vi "Incrementel Tester.vi"() -> ()   [LabVIEW 2013]
uses:
  <vilib>/Platform/TimedLoop/XDataNode/timing_clust.ctl
  <vilib>/Platform/TimedLoop/XDataNode/nitl_modes.ctl
  <vilib>/Platform/TimedLoop/XDataNode/wakeup.ctl
  <vilib>/rvi/Emulation/niFpgaSctlEmulationGetInTimedLoop.vi
  <vilib>/rvi/Emulation/niFpgaEmulationReportErrorSimple.vi
  <vilib>/rvi/Emulation/niFpgaGetClockAttributes.vi
  <vilib>/rvi/Emulation/niFpgaCriticalErrorInLSC.vi
  <vilib>/rvi/eio/common/nirviEmuTemplateMethod_errors.vi
  <vilib>/rvi/FIFO/Fifo_Resource/nirvififoEmulationWriteFpgaImpl.vi
  <vilib>/rvi/DataTransferAndStorage/Container/Common/niFpgaContainerGetUniqueNameForEmu.vi
  <vilib>/rvi/Emulation/niFpgaProcessEmulError.vi
  <vilib>/rvi/FIFO/Fifo_Resource/nirvififoEmulationReadFpgaImpl.vi
  LIDAR V2 Globals.vi
  <vilib>/Platform/TimedLoop/XDataNode/XDataNode.xnode
  <vilib>/eio/EIONode/EIONode.xnode
  <vilib>/rvi/DataTransferAndStorage/Container/XNode/niFpgaContainer.xnode
  <vilib>/rvi/FIFO/Fifo_Resource/nirvififoEmulationWrite.vi
  <vilib>/rvi/FIFO/Fifo_Resource/nirvififoEmulationRead.vi
  <vilib>/Platform/TimedLoop/XDataNode/XDNodeRunTimeDep.lvlib
panel:
  in  "PulseUpClck":u16=3
  in  "PulseWaitClck":u16=40
  in  "PFI2":bool
  in  "PFI3":bool
  in  "User Command Commit":bool
  in  "User Command":u8
  out "User Command Idle":bool
  out "User Command Status":u8
  in  "User Data 0":u8
  in  "User Data 1":u8
  out "User Error":bool
  out "Configured?":bool
  in  "MaxStartSample":u8
  out "PLL Locked":bool
  in  "AO Trig":bool
  in  "Devider":u8=3
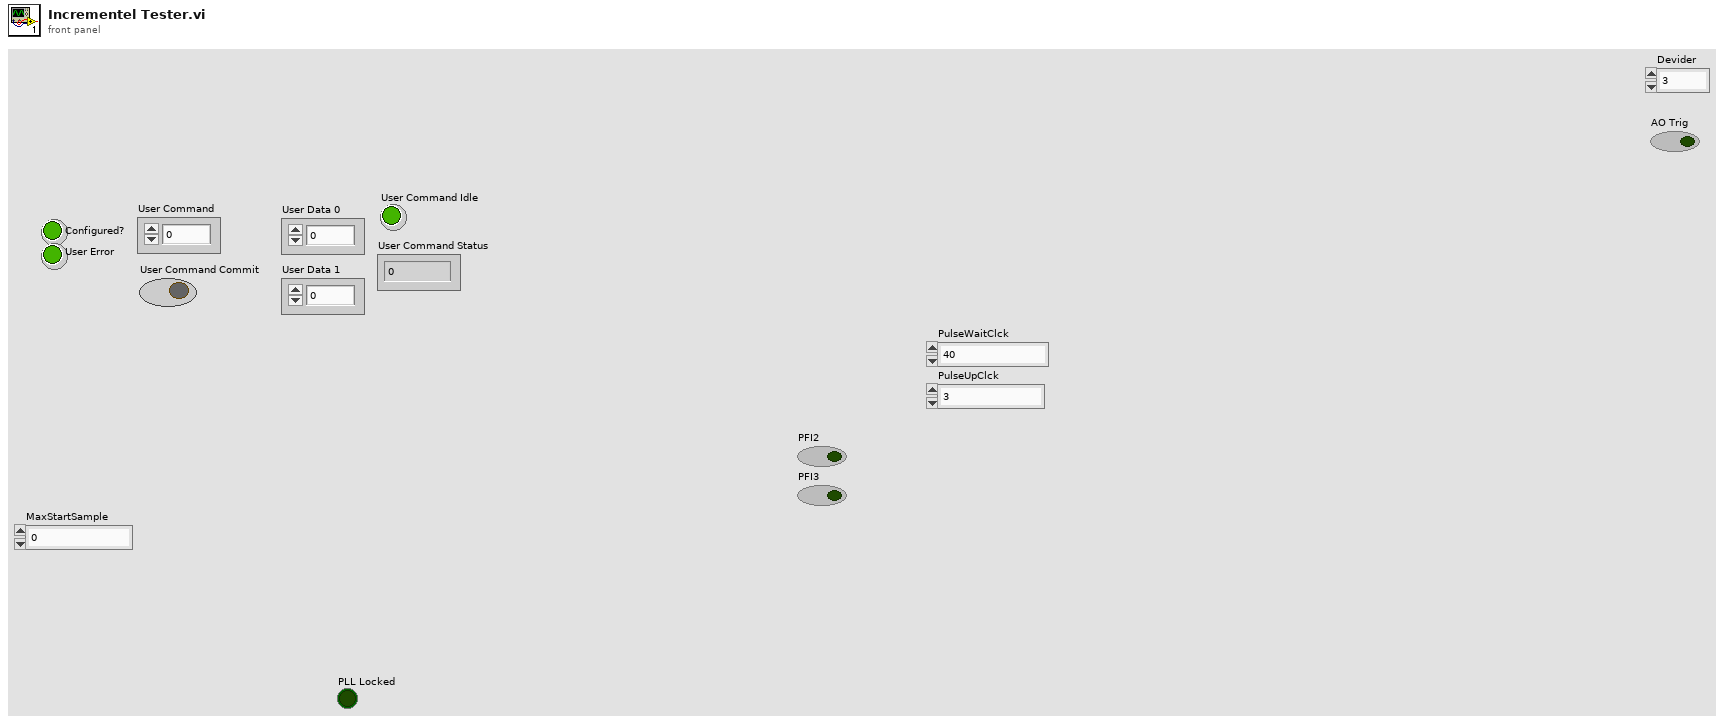
[diagram p1: front panel]
types:
  T1 = typedef "XDNodeRunTimeDep.lvlib/timing_clust.ctl" = cluster{"Expected End [f-1]":u64, "Actual End [f-1]":u64, "Finished Late? [f-1]":bool, "Expected End [i-1]":u64, "Actual End [i-1]":u64, "Finished Late? [i-1]":bool, "Expected Start [i]":u64, "Actual Start [i]":u64, "Expected Start [f]":u64, "Actual Start [f]":u64, "Source Name":string, "Structure Name":string, "Period":i64, "Deadline":i64, "Offset":i64, "Start":i64, "Priority":i32, "Timeout":i32, "Mode":T2, "Wakeup Reason":T3, "Error":errorcluster, "Source Type":string, "Secondary Source Type":string, "Global End Time":u64, "Global Start Time":u64, "Frame Duration":u64, "Iteration Duration":u64, "Assigned CPU":i32, "I/O Scan Engine Mode":u32}
  T2 = typedef "XDNodeRunTimeDep.lvlib/nitl_modes.ctl" = enum32{"No Change", "Process missed periods, maintain original phase", "Discard missed periods, maintain original phase", "Process missed periods, ignore original phase", "Discard missed periods, ignore original phase"}
  T3 = typedef "XDNodeRunTimeDep.lvlib/wakeup.ctl" = enum32{"Normal", "Aborted", "Asynchronous wakeup", "Timing source error", "Timed loop error", "Timeout"}
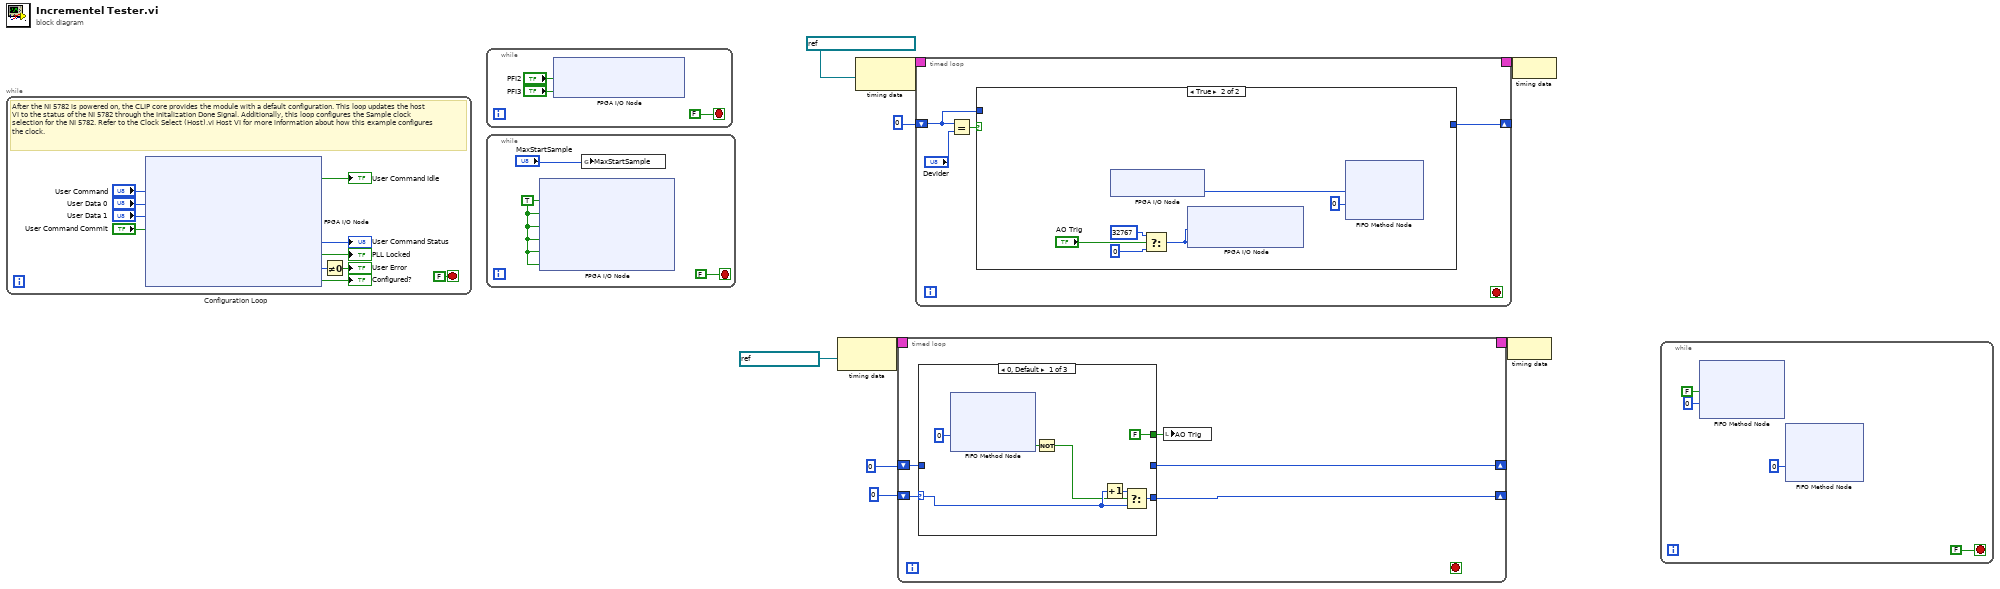
[diagram p0: block diagram]
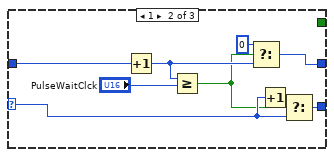
[diagram p2: hidden frame]
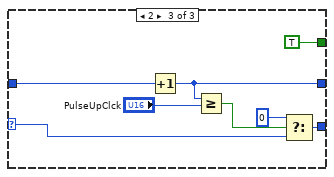
[diagram p3: hidden frame]
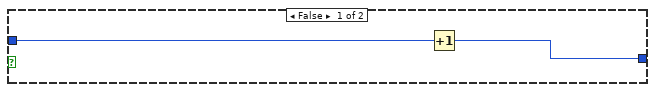
[diagram p4: hidden frame]
diagram:
  n1 = while "Configuration Loop" {
    stop <- FALSE stop-if-true
    # "After the NI 5782 is powered on, the CLIP core provides the module with a default configuration. This loop updates the host VI to the status of the NI 5782 through the Initalization Done Signal. Additionally, this loop configures the Sample clock selection for the NI 5782. Refer to the Clock Select (Host).vi Host VI for more information about how this example configures the clock."
    n2 = xnode "FPGA I/O Node"("IO Module\\User Command"="User Command", "IO Module\\User Data 0"="User Data 0", "IO Module\\User Data 1"="User Data 1", "IO Module\\User Command Commit"="User Command Commit") -> ("IO Module\\User Command Idle"=→"User Command Idle":bool, "IO Module\\User Command Status"=→"User Command Status":u8, "IO Module\\PLL Locked"=→"PLL Locked":bool, "IO Module\\User Error"=w14:u8, "IO Module\\Initialization Done"=→"Configured?":bool)  [unwired: 9 in, 9 out]
    n3 = Not Equal To 0?(x=w14) -> (x != 0?=→"User Error":bool)
  }
  n4 = while {
    stop <- FALSE stop-if-true
    n5 = xnode "FPGA I/O Node"("IO Module\\PFI 2 Wr Data"="PFI2", "IO Module\\PFI 3 Wr Data"="PFI3") -> ()  [unwired: 2 in, 2 out]
  }
  n6 = while {
    stop <- FALSE stop-if-true
    w25 = TRUE ("IO Module\\DIO Port 0 WE")
    n7 = xnode "FPGA I/O Node"("IO Module\\DIO Port 0 WE"=w25, "IO Module\\DIO Port 1 WE"=w25, "IO Module\\PFI 0 WE"=w25, "IO Module\\PFI 1 WE"=w25, "IO Module\\PFI 2 WE"=w25, "IO Module\\PFI 3 WE"=w25) -> ()  [unwired: 6 in, 6 out]
    n8 = global write "LIDAR V2 Globals.vi" "MaxStartSample"("MaxStartSample") -> ()
  }
  n9 = node-c288(refnum<k21> "100 MHz Clock" ("Source Name")) -> (w5:T1)
  n10 = node-c288(refnum<k21> "IO Module\\Data Clock" ("Source Name")) -> (w9:T1)
  n11 = timed-loop {
    timing: w5 -> [_]
    timing-out: [_] -> w4
    shift-right: [w30] -> _
    shift-left: i16 0 -> [w31]
    shift-right: [w28] -> _
    shift-left: u16 0 -> [w29]
    stop <- _ stop-if-true
    n12 = case shown="0, Default" w31 {
      selector: w31 -> [w37 w44 w50]
      tunnel: [w38 w45 w51] -> w30
      tunnel: w29 -> [_ w47 w55]
      tunnel: [_ w41 w54] -> w28
      tunnel: [FALSE _ TRUE] -> w27
      frame 0, Default {
        n13 = xnode ("FIFO Method Node")("Timeout"=0) -> ("Timed Out?"=w34:bool)  [unwired: 1 in, 2 out]
        n14 = Not(x=w34) -> (.not. x?=w32:bool)
        n15 = Increment(x=w37) -> (x+1=w36:i16)
        n16 = Select(t=w36, s=w32, f=w37) -> (s? t:f=w38:i16)
      }
      frame 1 {
        n17 = Increment(x=w47) -> (x+1=w42:u16)
        n18 = Greater Or Equal?(x=w42, y="PulseWaitClck") -> (x >= y?=w39:bool)
        n19 = Select(t=u16 0, s=w39, f=w42) -> (s? t:f=w41:u16)
        n20 = Increment(x=w44) -> (x+1=w43:i16)
        n21 = Select(t=w43, s=w39, f=w44) -> (s? t:f=w45:i16)
      }
      frame 2 {
        n22 = Increment(x=w55) -> (x+1=w54:u16)
        n23 = Greater Or Equal?(x=w54, y="PulseUpClck") -> (x >= y?=w52:bool)
        n24 = Select(t=i16 0, s=w52, f=w50) -> (s? t:f=w51:i16)
      }
    }
    n25 = local write "AO Trig"(w27) -> ()
  }
  n26 = timed-loop {
    timing: w9 -> [_]
    timing-out: [_] -> w8
    shift-right: [w59] -> _
    shift-left: u8 0 -> [w60]
    stop <- _ stop-if-true
    n27 = Equal?(x=w60, y="Devider") -> (x = y?=w58:bool)
    n28 = case shown="True" w58 {
      tunnel: w60 -> [w63 _]
      tunnel: [w62 _] -> w59
      frame False {
        n29 = Increment(x=w63) -> (x+1=w62:u8)
      }
      frame True {
        n30 = xnode "FPGA I/O Node"() -> ("IO Module\\AI 0"=w68:i16)  [unwired: 1 in, 1 out]
        n31 = Select(t=i16 32767 ("IO Module\\AO 0"), s="AO Trig", f=i16 0 ("IO Module\\AO 0")) -> (s? t:f=w67:i16)
        n32 = xnode "FPGA I/O Node"("IO Module\\AO 0 N-1"=w67, "IO Module\\AO 0 N"=w67) -> ()  [unwired: 2 in, 2 out]
        n33 = xnode ("FIFO Method Node")("Element"=w68, "Timeout"=0) -> ()  [unwired: 1 in, 2 out]
      }
    }
  }
  n34 = node-c288(w4) -> ()
  n35 = node-c288(w8) -> ()
  n36 = while {
    stop <- FALSE stop-if-true
    n37 = xnode ("FIFO Method Node")("Element"=FALSE, "Timeout"=0) -> ()  [unwired: 1 in, 2 out]
    n38 = xnode ("FIFO Method Node")("Timeout"=0) -> ()  [unwired: 1 in, 3 out]
  }
